vi "Servo Sine wave.vi"(7 "Theshold":u32=10, 8 "Positions":dbl[](array[numeric]) min=-179.9 max=179.9, 9 "Acceleration_profile":u32=20, 10 "Velocity_profile":u32=10, 11 "Com port":refnum<visa-resource-name> caption="instrument handle") -> (2 "dynamixel_error":string, 3 "dynamixel_comm_result":string)   [LabVIEW 2022 SP3]
uses:
  Library/dxl_x64_c.lvlib
  <vilib>/ptbypt/NI_PtbyPt.lvlib
panel:
  out "Waveform Chart":cluster{dbl, "function return":u32}(graph)
  out "Numeric":dbl
  in  "Time of Sine Wave":dbl=1.0
  in  "Frequency of Sine Wave":dbl=1.0
  in  "Sine Wave Max Angle":dbl=10.0
  out "Approx Move time (ms)":u32
  in  "ADDR_Theshold":u16=24
  in  "ADDR_Acceleration_profile":u16=108
  in  "ADDR_Velocity_profile":u16=112
  in  "Terminate Initally Position":bool
  out "value : PRO (knob)\npresent position":u32(knob) scale=150000.0..-150000.0
  in  "Max_position_limit_value":u32=4095
  in  "ADDR_Max_Position_Limit":u16=48
  in  "ADDR_PRO_\nPRESENT_POSITION":u16=132
  in  "ADDR_PRO_\nGOAL_POSITION":u16=116
  in  "ADDR_PRO_\nTORQUE_ENABLE":u16=64
  in  "protocol_version":i32=2
  out "port_num":i32
  in  "dynamixel_id":u8=1
  in  "baud_rate":i32=57600
  # "Available Dynamixel model on this example : All models using Protocol 2.0\nThis example is designed for using a Dynamixel PRO 54-200, and an USB2DYNAMIXEL.\nTo use another Dynamixel model, such as X series, see their details in E-Manual(support.robotis.com) \n   and edit \"numeric control\"s seen left with \"Edit Text\" tool.\nBe sure that Dynamixel PRO properties are already set as %% ID : 1 / Baudnum : 1 (Baudrate : 57600)\n\n1. Run example by click above \"Run\" button (below \"Edit\" menu).\n2. Drag \"dial\" then you may see the Dynamixel and \"knob\" rotating\n3. To finish the example, press \"terminate\" button."
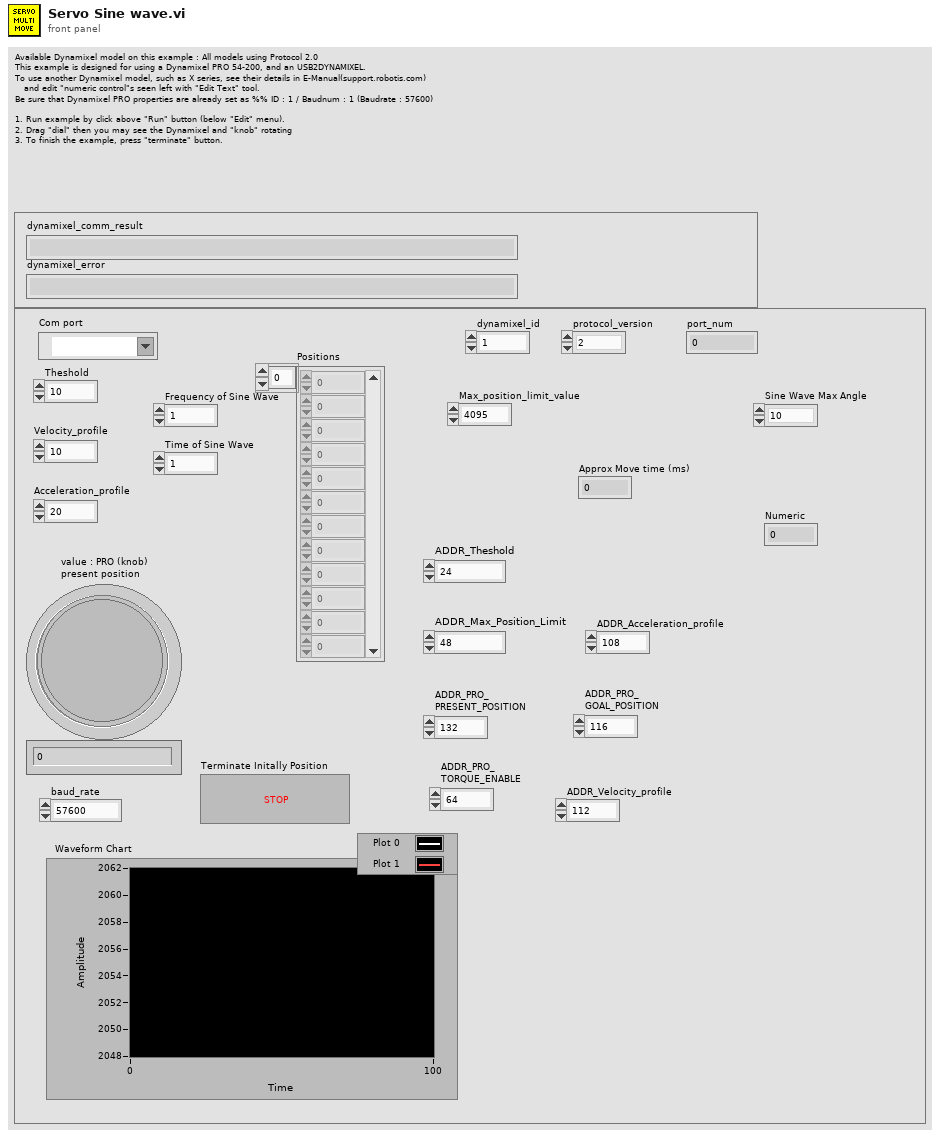
[diagram p1: front panel]
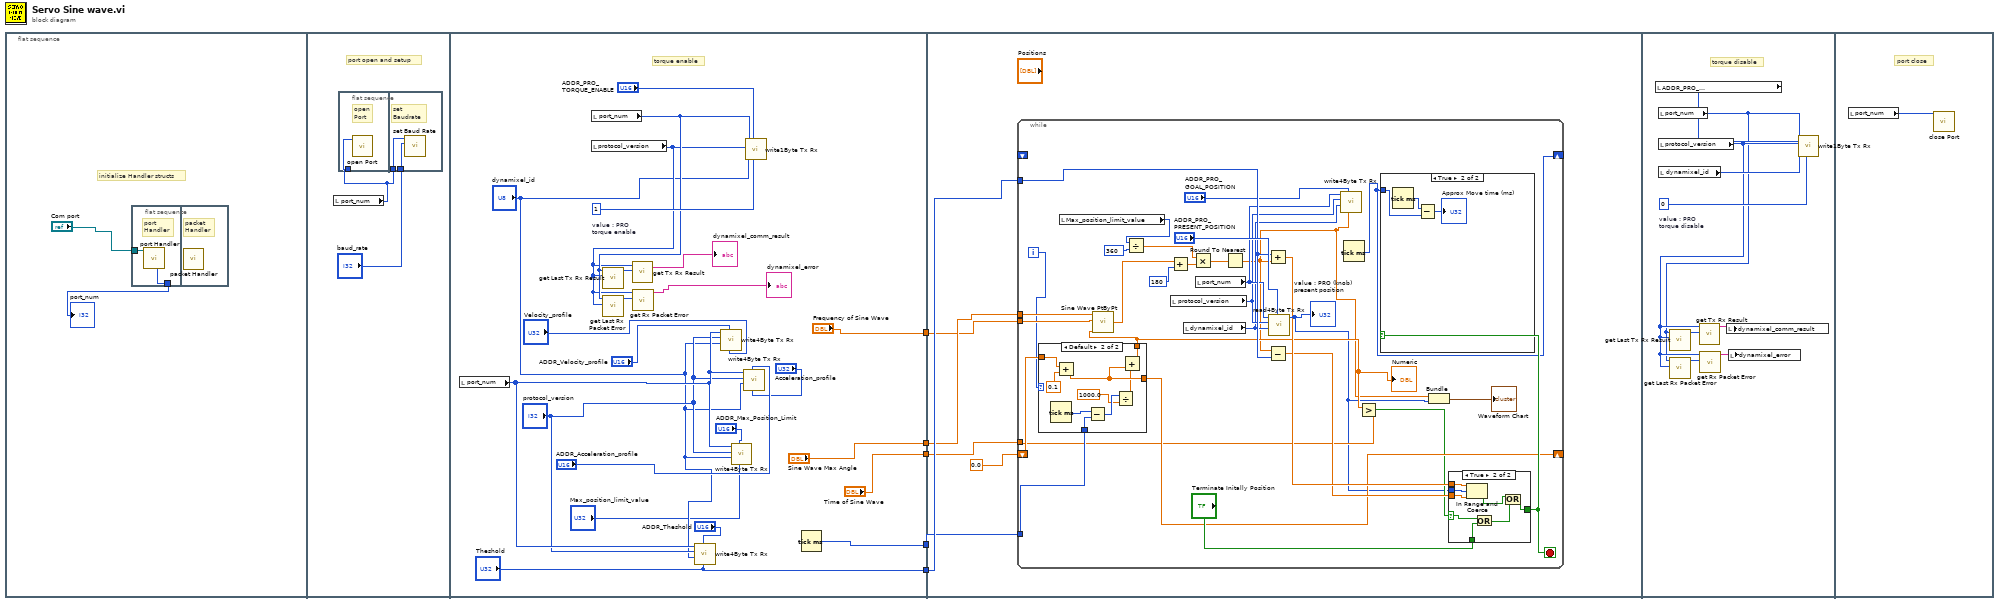
[diagram p0: block diagram]
diagram:
  n1 = flat-sequence {
    tunnel: ["Theshold"] -> w5
    tunnel: ["Sine Wave Max Angle"] -> w4
    tunnel: [w17] -> w3
    tunnel: ["Frequency of Sine Wave"] -> w2
    tunnel: ["Time of Sine Wave"] -> w1
    tunnel: w5 -> [w43]
    tunnel: w4 -> [w42]
    tunnel: w3 -> [w41]
    tunnel: w2 -> [w39]
    tunnel: w1 -> [w38]
    frame #0 {
      # "initialize Handler structs"
      n2 = flat-sequence {
        tunnel: [w9] -> w7
        tunnel: "Com port" -> [w8]
        frame #0 {
          # "port\nHandler"
          n3 = call "port Handler.vi"("port_name"=w8) -> ("function return"=w9:i32)  [unwired: 9 in, 1 out]
        }
        frame #1 {
          # "packet\nHandler"
          n4 = call "packet Handler.vi"() -> ()  [unwired: 11 in, 1 out]
        }
      }
      "port_num" <- w7
    }
    frame #1 {
      # "port open and setup"
      n5 = local read "port_num"() -> (w11:i32)
      n6 = flat-sequence {
        tunnel: w11 -> [w12]
        tunnel: w11 -> [w14]
        tunnel: "baud_rate" -> [w13]
        frame #0 {
          # "open\nPort"
          n7 = call "open Port.vi"("port_num"=w12) -> ()  [unwired: 9 in, 2 out]
        }
        frame #1 {
          # "set\nBaudrate"
          n8 = call "set Baud Rate.vi"("baudrate"=w13, "port_num"=w14) -> ()  [unwired: 8 in, 2 out]
        }
      }
    }
    frame #2 {
      w37 = 1  # value : PRO torque enable
      # "torque enable"
      n9 = local read "port_num"() -> (w27:i32)
      n10 = local read "protocol_version"() -> (w33:i32)
      n11 = local read "port_num"() -> (w34:i32)
      n12 = call "get Last Tx Rx Result.vi"("protocol_version"=w33, "port_num"=w34) -> ("function return"=w36:i32)  [unwired: 8 in, 1 out]
      n13 = call "get Last Rx Packet Error.vi"("protocol_version"=w33, "port_num"=w34) -> ("function return"=w35:u8)  [unwired: 8 in, 1 out]
      n14 = call "get Tx Rx Result.vi"("result"=w36, "protocol_version"=w33) -> ("function return"=→"dynamixel_comm_result":string)  [unwired: 8 in, 1 out]
      n15 = call "get Rx Packet Error.vi"("error"=w35, "protocol_version"=w33) -> ("function return"=→"dynamixel_error":string)  [unwired: 8 in, 1 out]
      n16 = call "write4Byte Tx Rx.vi"("data"="Theshold", "address"="ADDR_Theshold", "id"="dynamixel_id", "protocol_version"="protocol_version", "port_num"=w27) -> ()  [unwired: 6 in, 1 out]
      n17 = call "write4Byte Tx Rx.vi"("data"="Velocity_profile", "address"="ADDR_Velocity_profile", "id"="dynamixel_id", "protocol_version"="protocol_version", "port_num"=w27) -> ()  [unwired: 6 in, 1 out]
      n18 = call "write4Byte Tx Rx.vi"("data"="Max_position_limit_value", "address"="ADDR_Max_Position_Limit", "id"="dynamixel_id", "protocol_version"="protocol_version", "port_num"=w27) -> ()  [unwired: 6 in, 1 out]
      n19 = call "write4Byte Tx Rx.vi"("data"="Acceleration_profile", "address"="ADDR_Acceleration_profile", "id"="dynamixel_id", "protocol_version"="protocol_version", "port_num"=w27) -> ()  [unwired: 6 in, 1 out]
      n20 = call "write1Byte Tx Rx.vi"("data"=w37, "address"="ADDR_PRO_\nTORQUE_ENABLE", "id"="dynamixel_id", "protocol_version"=w33, "port_num"=w34) -> ()  [unwired: 6 in, 1 out]
      n21 = Tick Count (ms)() -> (millisecond timer value=w17:u32)
    }
    frame #3 {
      n22 = while {
        tunnel: w43 -> [w63]
        shift-right: [w57] -> _
        shift-left: _ -> [_]
        tunnel: w42 -> [w56]
        tunnel: w41 -> [w55]
        shift-right: [w52] -> _
        shift-left: 0.0 -> [w53]
        tunnel: w39 -> [w51]
        tunnel: w38 -> [w50]
        i -> [w48]
        stop <- w62 stop-if-true
        n23 = case shown="Default" w48 {
          tunnel: w55 -> [_ w82]
          tunnel: w53 -> [w74 w81]
          tunnel: [w74 w79] -> w52
          tunnel: [w74 w78] -> w47
          frame 0 {
          }
          frame Default {
            n24 = Tick Count (ms)() -> (millisecond timer value=w83:u32)
            n25 = Add(x=w81, y=0.1 ("Numeric")) -> (x+y=w79:dbl)
            n26 = Subtract(x=w83, y=w82) -> (x-y=w76:u32)
            n27 = Divide(x=w76, y=1000.0) -> (x/y=w77:dbl)
            n28 = Add(x=w77, y=w79) -> (x+y=w78:dbl)
          }
        }
        "Numeric" <- w47
        n29 = local read "Max_position_limit_value"() -> (w70:u32)
        n30 = call <vilib>:"Sine Wave PtByPt.vi"("time"=w47, "frequency"=w51, "amplitude"=w56) -> ("sine wave"=w54:dbl)  [unwired: 1 in]
        n31 = Divide(x=w70, y=360) -> (x/y=w68:dbl)
        n32 = Add(x=w54, y=180) -> (x+y=w65:dbl)
        n33 = local read "protocol_version"() -> (w59:i32)
        n34 = local read "dynamixel_id"() -> (w58:u8)
        n35 = Multiply(x=w68, y=w65) -> (x*y=w67:dbl)
        n36 = local read "port_num"() -> (w60:i32)
        n37 = Round To Nearest(number=w67) -> (nearest integer value=w46:dbl)
        n38 = Add(x=w63, y=w46) -> (x+y=w73:dbl)
        n39 = Subtract(x=w46, y=w63) -> (x-y=w72:dbl)
        n40 = call "read4Byte Tx Rx.vi"("address"="ADDR_PRO_\nPRESENT_POSITION", "id"=w58, "protocol_version"=w59, "port_num"=w60) -> ("function return"=w45:u32)  [unwired: 6 in, 1 out]
        "value : PRO (knob)\npresent position" <- w45
        n41 = call "write4Byte Tx Rx.vi"("data"=w46, "address"="ADDR_PRO_\nGOAL_POSITION", "id"=w58, "protocol_version"=w59, "port_num"=w60) -> ()  [unwired: 6 in, 1 out]
        n42 = Tick Count (ms)() -> (millisecond timer value=w57:u32)
        n43 = Greater?(x=w47, y=w50) -> (0:w49:bool)
        n44 = Bundle(w46, "function return"=w45) -> (→"Waveform Chart":cluster{dbl, "function return":u32})  [unwired: 1 in]
        n45 = case shown="True" w49 {
          selector: w49 -> [_ w87]
          tunnel: w73 -> [_ w92]
          tunnel: w72 -> [_ w91]
          tunnel: w45 -> [_ w90]
          tunnel: "Terminate Initally Position" -> [w84 w86]
          tunnel: [w84 w88] -> w62
          frame False {
          }
          frame True {
            n46 = In Range and Coerce(upper limit=w92, x=w90, lower limit=w91) -> (In Range?=w89:bool)  [unwired: 1 out]
            n47 = Or(x=w87, y=w86) -> (x .or. y?=w85:bool)
            n48 = Or(x=w89, y=w85) -> (x .or. y?=w88:bool)
          }
        }
        n49 = case shown="True" w62 {
          tunnel: w57 -> [_ w94]
          frame False {
          }
          frame True {
            n50 = Tick Count (ms)() -> (millisecond timer value=w95:u32)
            n51 = Subtract(x=w95, y=w94) -> (x-y=→"Approx Move time (ms)":u32)
          }
        }
      }
    }
    frame #4 {
      w103 = 0  # value : PRO torque disable
      # "torque disable"
      n52 = local read "ADDR_PRO_\nTORQUE_ENABLE"() -> (w102:u16)
      n53 = local read "port_num"() -> (w98:i32)
      n54 = local read "protocol_version"() -> (w99:i32)
      n55 = local read "dynamixel_id"() -> (w104:u8)
      n56 = call "get Last Tx Rx Result.vi"("protocol_version"=w99, "port_num"=w98) -> ("function return"=w100:i32)  [unwired: 8 in, 1 out]
      n57 = call "get Last Rx Packet Error.vi"("protocol_version"=w99, "port_num"=w98) -> ("function return"=w101:u8)  [unwired: 8 in, 1 out]
      n58 = call "get Tx Rx Result.vi"("result"=w100, "protocol_version"=w99) -> ("function return"=w97:string)  [unwired: 8 in, 1 out]
      n59 = call "get Rx Packet Error.vi"("error"=w101, "protocol_version"=w99) -> ("function return"=w96:string)  [unwired: 8 in, 1 out]
      n60 = local write "dynamixel_comm_result"(w97) -> ()
      n61 = local write "dynamixel_error"(w96) -> ()
      n62 = call "write1Byte Tx Rx.vi"("data"=w103, "address"=w102, "id"=w104, "protocol_version"=w99, "port_num"=w98) -> ()  [unwired: 6 in, 1 out]
    }
    frame #5 {
      # "port close"
      n63 = local read "port_num"() -> (w105:i32)
      n64 = call "close Port.vi"("port_num"=w105) -> ()  [unwired: 10 in, 1 out]
    }
  }
